vi "Write output state.vi"(8 "error in (no error)":errorcluster, 10 "output state (Constant Voltage)":i32(ring) items=["Constant Voltage"=0, "Constant Current"=1, "Unregulated"=4, "Over Voltage"=2, "Over Current"=3], 11 "Query Output State Msg in":refnum<class "Query Output State Msg.lvclass">) -> (0 "error out":errorcluster, 3 "Query Output State Msg out":refnum<class "Query Output State Msg.lvclass">)   [LabVIEW 2013, in "CS++DCPwr.lvlib" / "Query Output State Msg.lvclass"]
uses:
  Query Output State Msg.lvclass
  Query Output State Msg.lvclass/Query Output State Msg.ctl
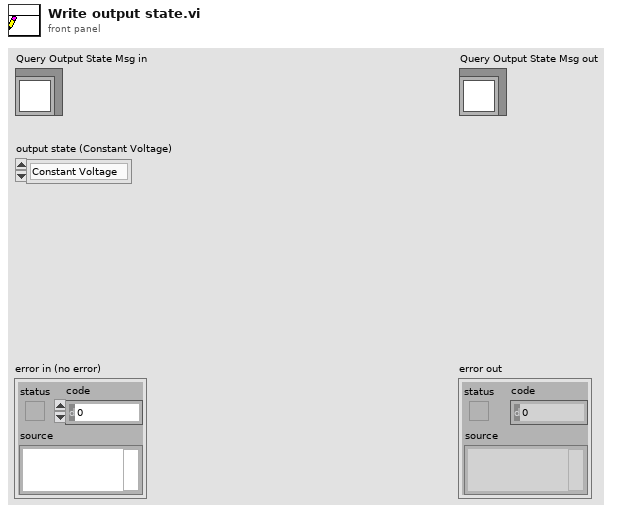
[diagram p1: front panel]
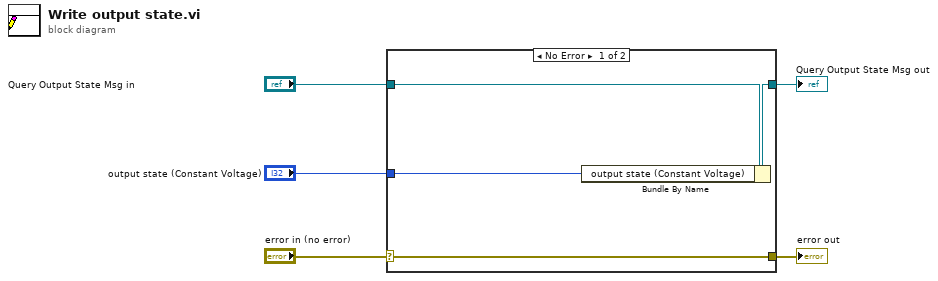
[diagram p0: block diagram]
diagram:
  n1 = case shown="No Error" "error in (no error)" {
    selector: "error in (no error)" -> [w9 w10]
    tunnel: [w9 w10] -> w4
    tunnel: [w7 w11] -> w2
    tunnel: "Query Output State Msg in" -> [w8 w11]
    tunnel: "output state (Constant Voltage)" -> [w6 _]
    frame No Error {
      n2 = Bundle By Name(cluster=w8, "output state (Constant Voltage)"=w6) -> (w7:refnum<class "Query Output State Msg.lvclass">)
    }
    frame Error {
    }
  }
  "error out" <- w4
  "Query Output State Msg out" <- w2
